vi "Preview Index.vi"(8 "error in (no error)":errorcluster, 11 "CO2 Actor in":refnum<class "CO2 Actor.lvclass">) -> (0 "error out":errorcluster, 2 "Index":i32=-1, 3 "CO2 Actor out":refnum<class "CO2 Actor.lvclass">)   [LabVIEW 2015, in "cRIO-Carbondioxide.lvlib" / "CO2-Actor.lvlib" / "CO2 Actor.lvclass"]
uses:
  CO2 Actor.lvclass
  CO2 Actor.lvclass/CO2 Actor.ctl
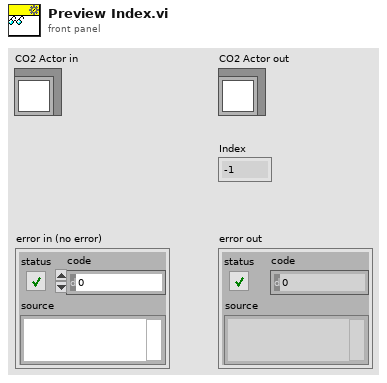
[diagram p1: front panel]
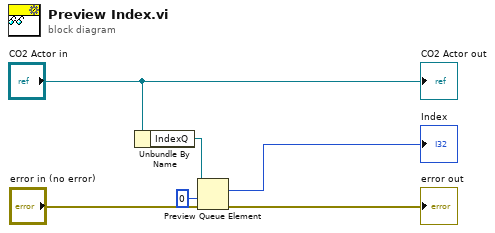
[diagram p0: block diagram]
diagram:
  n1 = Unbundle By Name("CO2 Actor in") -> ("IndexQ"=w4:refnum<queue>)
  n2 = Preview Queue Element(queue=w4, timeout in ms (-1)=0, error in (no error)="error in (no error)") -> (element=→"Index":i32, error out=→"error out":errorcluster)  [unwired: 2 out]
  "CO2 Actor out" <- "CO2 Actor in"
